vi "DSF.Engine.Plugin.Set Rx Transfer Groups.vi"(10 "Rx Transfer Groups":refnum<class "DSF.Engine.Transfer Group.lvclass">[](array[class]), 11 "Plugin in":refnum<class "Plugin.lvclass">) -> (3 "Plugin out":refnum<class "Plugin.lvclass">)   [LabVIEW 2016, in "DSF.Engine.lvlib" / "Plugin.lvclass"]
uses:
  Plugin.lvclass
  Transfer/DSF.Engine.Transfer Group.lvclass
  Plugin.lvclass/Plugin.ctl
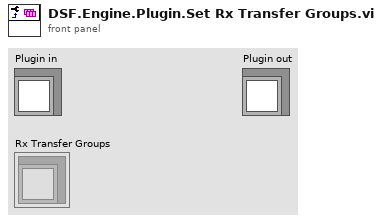
[diagram p1: front panel]
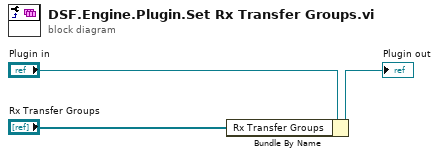
[diagram p0: block diagram]
diagram:
  n1 = Bundle By Name(cluster="Plugin in", "Rx Transfer Groups"="Rx Transfer Groups") -> (→"Plugin out":refnum<class "Plugin.lvclass">)
